vi "Update Save Pressed.vi"(8 "error in (no error)":errorcluster, 11 "Map Model in":refnum<class "Map Model.lvclass">) -> (0 "error out":errorcluster, 3 "Map Model out":refnum<class "Map Model.lvclass">)   [LabVIEW 2020, in "Map Model.lvlib" / "Map Model.lvclass"]
uses:
  Map Model.lvclass
  Map Model.lvclass/Map Model.ctl
  Stack/Stack.lvclass
panel:
  # "NOTICE -- YOU MUST LEAVE THIS NOTICE IN PLACE.\n\nCopyright (c) 2017, LIANG LIU Shawn.Liu.cn@gmail.com\nAll rights reserved.\n\nRedistribution and use in source and binary forms, with or without modification, are permitted provided that the following conditions are met:\n-Redistributions of source code must retain the above copyright notice, this list of conditions and the following disclaimer.\n-Redistributions in binary form must reproduce the above copyright notice, this list of conditions and the following disclaimer in the documentation and/or other materials provided with the distribution.\n-Neither the name of the eLp nor the names of its contributors may be used to endorse or promote products derived from this software without specific prior written permission.\n\nTHIS SOFTWARE IS PROVIDED BY THE COPYRIGHT HOLDERS AND CONTRIBUTORS \"AS IS\" AND ANY EXPRESS OR IMPLIED WARRANTIES, INCLUDING, BUT NOT LIMITED TO, THE IMPLIED WARRANTIES OF MERCHANTABILITY AND FITNESS FOR A PARTICULAR PURPOSE ARE DISCLAIMED. IN NO EVENT SHALL THE COPYRIGHT HOLDER OR CONTRIBUTORS BE LIABLE FOR ANY DIRECT, INDIRECT, INCIDENTAL, SPECIAL, EXEMPLARY, OR CONSEQUENTIAL DAMAGES (INCLUDING, BUT NOT LIMITED TO, PROCUREMENT OF SUBSTITUTE GOODS OR SERVICES; LOSS OF USE, DATA, OR PROFITS; OR BUSINESS INTERRUPTION) HOWEVER CAUSED AND ON ANY THEORY OF LIABILITY, WHETHER IN CONTRACT, STRICT LIABILITY, OR TORT (INCLUDING NEGLIGENCE OR OTHERWISE) ARISING IN ANY WAY OUT OF THE USE OF THIS SOFTWARE, EVEN IF ADVISED OF THE POSSIBILITY OF SUCH DAMAGE."
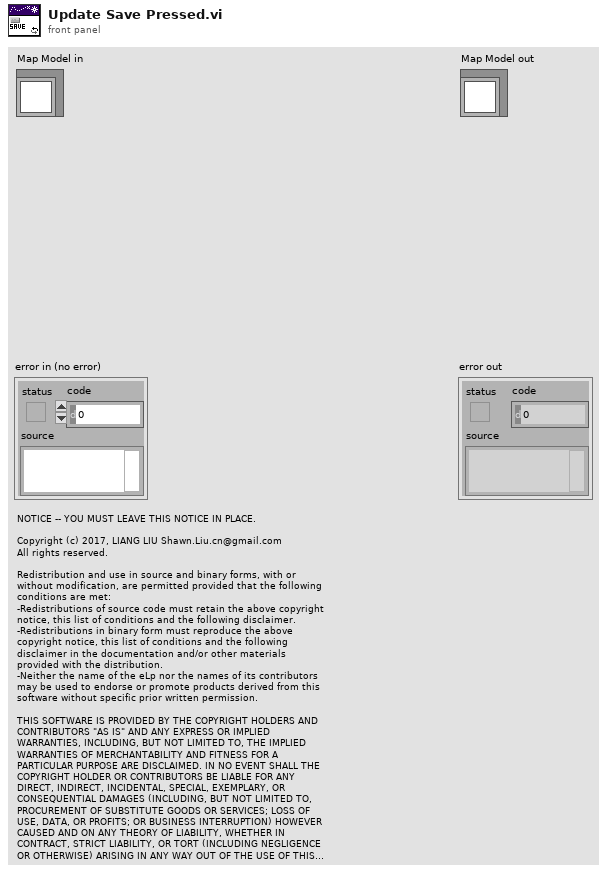
[diagram p1: front panel]
types:
  T1 = enum8{"Enabled", "Disabled", "Disabled and Grayed Out"}
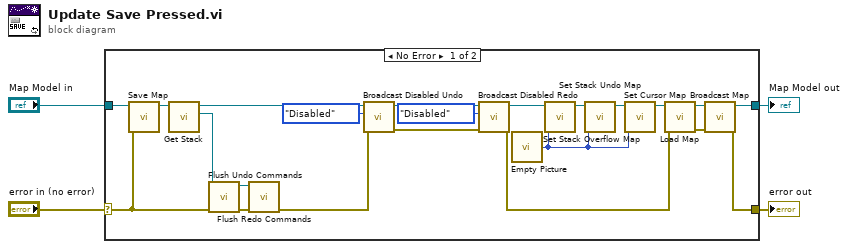
[diagram p0: block diagram]
diagram:
  n1 = case shown="No Error" "error in (no error)" {
    selector: "error in (no error)" -> [w23 w28]
    tunnel: "Map Model in" -> [w26 w27]
    tunnel: [w25 w28] -> w3
    tunnel: [w24 w27] -> w2
    frame No Error {
      n2 = call "Save Map.vi"("error in (no error)"=w23, "Map Model in"=w26) -> ("Map Model out"=w16:refnum<class "Map Model.lvclass">)  [unwired: 8 in, 1 out]
      n3 = call "Get Stack.vi"("Map Model in"=w16) -> ("Stack"=w13:refnum<class "Stack.lvclass">, "Map Model out"=w9:refnum<class "Map Model.lvclass">)  [unwired: 9 in]
      n4 = call "Flush Undo Commands.vi"("error in (no error)"=w23, "Stack in"=w13) -> ("error out"=w15:errorcluster, "Stack out"=w14:refnum<class "Stack.lvclass">)  [unwired: 8 in]
      n5 = call "Flush Redo Commands.vi"("error in (no error)"=w15, "Stack in"=w14) -> ("error out"=w7:errorcluster)  [unwired: 8 in, 1 out]
      n6 = call "Broadcast Disabled Undo.vi"("error in (no error)"=w7, "Disabled Undo"=T1."Disabled", "Map Model in"=w9) -> ("error out"=w8:errorcluster, "Map Model out"=w12:refnum<class "Map Model.lvclass">)  [unwired: 7 in]
      n7 = call "Broadcast Disabled Redo.vi"("error in (no error)"=w8, "Disabled Redo"=T1."Disabled", "Map Model in"=w12) -> ("error out"=w6:errorcluster, "Map Model out"=w5:refnum<class "Map Model.lvclass">)  [unwired: 7 in]
      n8 = call "Empty Picture"() -> ("empty picture"=w17:picture)
      n9 = call "Set Stack Overflow Map.vi"("Stack Overflow Map"=w17, "Map Model in"=w5) -> ("Map Model out"=w20:refnum<class "Map Model.lvclass">)  [unwired: 9 in]
      n10 = call "Set Stack Undo Map.vi"("Stack Undo Map"=w17, "Map Model in"=w20) -> ("Map Model out"=w19:refnum<class "Map Model.lvclass">)  [unwired: 9 in]
      n11 = call "Set Cursor Map.vi"("Cursor Map"=w17, "Map Model in"=w19) -> ("Map Model out"=w18:refnum<class "Map Model.lvclass">)  [unwired: 9 in]
      n12 = call "Load Map.vi"("error in (no error)"=w6, "Map Model in"=w18) -> ("error out"=w21:errorcluster, "Map Model out"=w22:refnum<class "Map Model.lvclass">)  [unwired: 8 in]
      n13 = call "Broadcast Map.vi"("error in (no error)"=w21, "Map Model in"=w22) -> ("error out"=w25:errorcluster, "Map Model out"=w24:refnum<class "Map Model.lvclass">)  [unwired: 8 in]
    }
    frame Error {
    }
  }
  "error out" <- w3
  "Map Model out" <- w2
